vi "Set Sensor Menus.vi"(8 "Error In":errorcluster, 11 "ListBox Refs":refnum<vi>[](array[refnum])) -> (0 "Error Out":errorcluster)   [LabVIEW 2021]
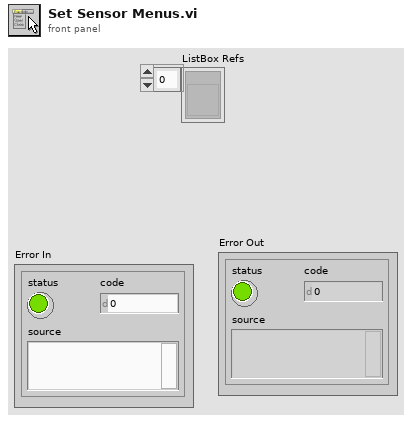
[diagram p1: front panel]
types:
  T1 = enum16{"None", "On Hover", "On Key Focus", "On Hover or Key Focus"}
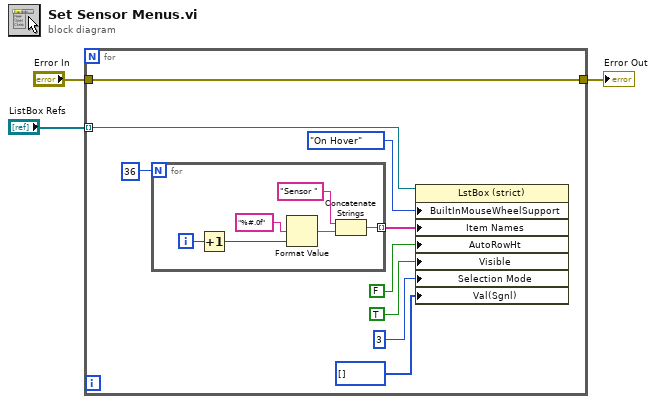
[diagram p0: block diagram]
diagram:
  n1 = for {
    tunnel: "ListBox Refs" -> [w11] mode=indexing
    tunnel: "Error In" -> [w8]
    tunnel: [w8] -> w2
    n2 = for {
      N: 36 -> [_]
      tunnel: [w14] -> w9 mode=indexing
      i -> [w17]
      n3 = Increment(x=w17) -> (x+1=w16:i32)
      n4 = Format Value(format string="%#.0f", value (0)=w16) -> (output string=w15:string)  [unwired: 1 in]
      n5 = Concatenate Strings("Sensor ", w15) -> (w14:string)
    }
    n6 = property on="Property Node" class="LstBox (strict)"(reference=w11, "BuiltInMouseWheelSupport"=T1."On Hover" ("Built-In Mouse Wheel Support"), "Item Names"=w9, "AutoRowHt"=FALSE ("Autosizing Row Height"), "Visible"=TRUE, "Selection Mode"=3, "Val(Sgnl)"=i32[] [] ("Value")) -> ()  [unwired: 1 in, 2 out]
  }
  "Error Out" <- w2
